vi "Test_QueueTransport_ValueOK.vi"(8 "error in (no error)":errorcluster, 11 "TestCase in":refnum<class "TestTransport.lvclass">) -> (0 "error out":errorcluster, 3 "TestCase out":refnum<class "TestTransport.lvclass">)   [LabVIEW 2015, in "Transport.lvlib" / "TestTransport.lvclass"]
uses:
  TestTransport.lvclass
  QueueTransport/QueueTransport.lvclass/QueueTransport.ctl
  <vilib>/Utility/error.llb/Error Cluster From Error Code.vi
  QueueTransport/QueueTransport.lvclass
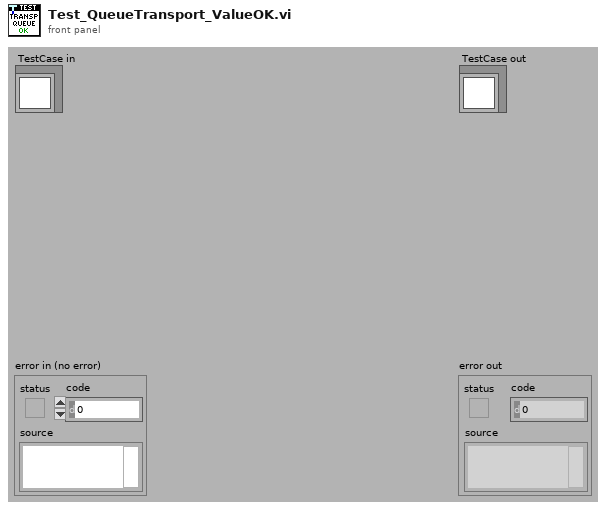
[diagram p1: front panel]
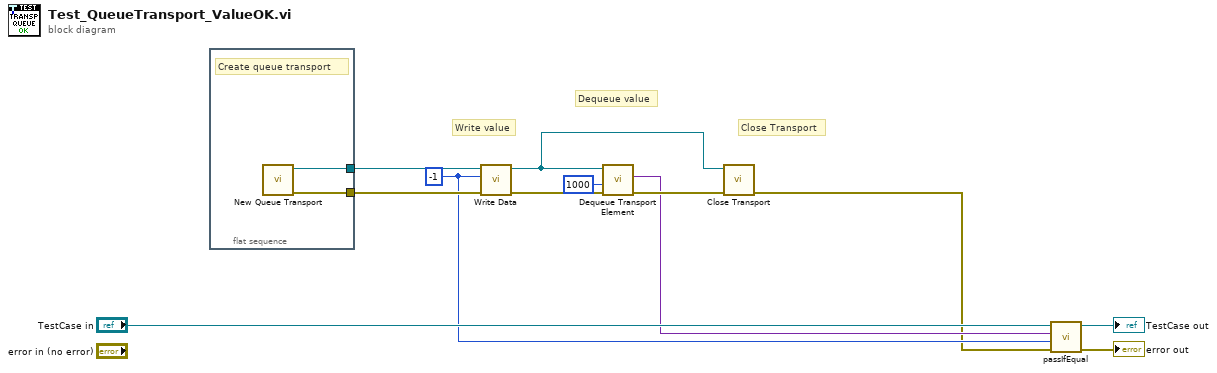
[diagram p0: block diagram]
diagram:
  w3 = -1
  # "Close Transport"
  # "Write value"
  # "Dequeue value"
  n1 = flat-sequence {
    tunnel: [w14] -> w9
    tunnel: [w13] -> w8
    frame #0 {
      # "Create queue transport"
      n2 = call "New Queue Transport.vi"() -> ("error out"=w13:errorcluster, "QueueTransport"=w14:refnum<class "QueueTransport.lvclass">)  [unwired: 10 in]
    }
  }
  n3 = call-dynamic "Write Data.vi"("error in (no error)"=w8, "Value"=w3, "QueueTransport In"=w9) -> ("error out"=w7:errorcluster, "QueueTransport Out"=w1:refnum<class "QueueTransport.lvclass">)  [unwired: 7 in]
  n4 = call "Dequeue Transport Element.vi"("error in (no error)"=w7, "Timeout In ms (-1)"=1000, "QueueTransport in"=w1) -> ("error out"=w6:errorcluster, "Data"=w4:variant)  [unwired: 5 in, 2 out]
  n5 = call-dynamic "Close Transport.vi"("error in (no error)"=w6, "QueueTransport in"=w1) -> ("error out"=w2:errorcluster)  [unwired: 9 in]
  n6 = call-dynamic "passIfEqual.vi"("error in (no error)"=w2, "y"=w3, "x"=w4, "TestCase in"="TestCase in") -> ("error out"=→"error out":errorcluster, "TestCase out"=→"TestCase out":refnum<class "TestTransport.lvclass">)  [unwired: 6 in]
